vi "is_roi_inside_roi.vi"(8 "Error In":errorcluster, 10 "ROI Outer":T1, 11 "ROI Inner":T1) -> (0 "Error Out":errorcluster, 3 "Inner is inside Outer":bool)   [LabVIEW 2019]
doc: "Determines if one ROI is inside another ROI or not based on their global rectangles."
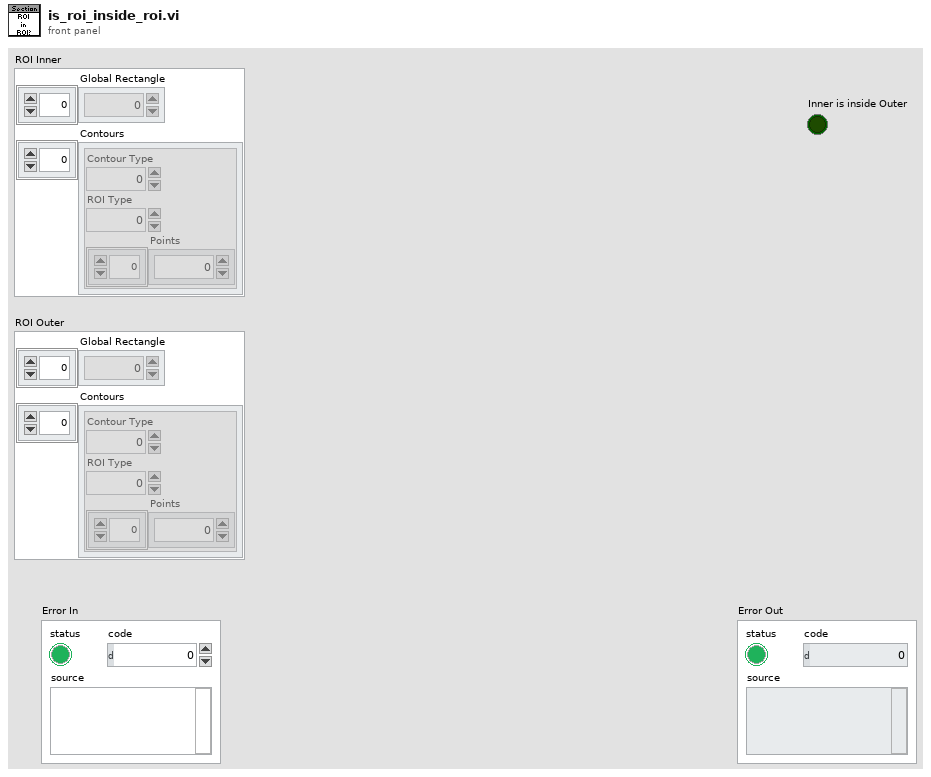
[diagram p1: front panel]
types:
  T1 = cluster{"Global Rectangle":i32[], "Contours":cluster{"Contour Type":u32, "ROI Type":u32, "Points":i32[]}[]}
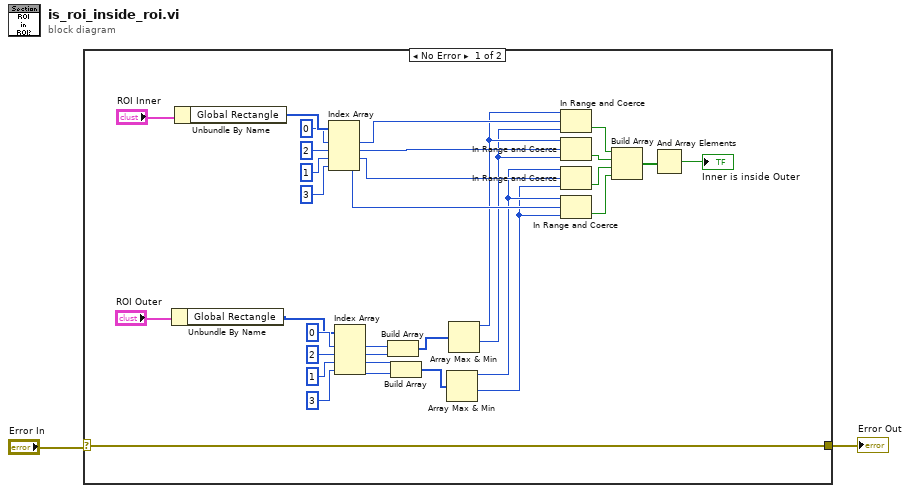
[diagram p0: block diagram]
diagram:
  n1 = case shown="No Error" "Error In" {
    selector: "Error In" -> [w35 w36]
    tunnel: [w35 w36] -> w1
    frame No Error {
      n2 = Unbundle By Name("ROI Outer") -> ("Global Rectangle"=w24:i32[])
      n3 = Unbundle By Name("ROI Inner") -> ("Global Rectangle"=w32:i32[])
      n4 = Index Array(array=w32, index #1=0 ("index"), index #2=2 ("index"), index #3=1 ("index"), index #4=3 ("index")) -> (element #1=w18:i32, element #2=w17:i32, element #3=w16:i32, element #4=w15:i32)
      n5 = Index Array(array=w24, index #1=0 ("index"), index #2=2 ("index"), index #3=1 ("index"), index #4=3 ("index")) -> (element #1=w19:i32, element #2=w22:i32, element #3=w21:i32, element #4=w20:i32)
      n6 = Build Array(w19, w22) -> (w14:i32[])
      n7 = Build Array(w21, w20) -> (w13:i32[])
      n8 = Array Max & Min(array=w13) -> (max value=w10:i32, min value=w9:i32)  [unwired: 2 out]
      n9 = Array Max & Min(array=w14) -> (max value=w12:i32, min value=w11:i32)  [unwired: 2 out]
      n10 = In Range and Coerce(upper limit=w12, x=w18, lower limit=w11) -> (In Range?=w8:bool)  [unwired: 1 out]
      n11 = In Range and Coerce(upper limit=w12, x=w17, lower limit=w11) -> (In Range?=w7:bool)  [unwired: 1 out]
      n12 = In Range and Coerce(upper limit=w10, x=w16, lower limit=w9) -> (In Range?=w6:bool)  [unwired: 1 out]
      n13 = In Range and Coerce(upper limit=w10, x=w15, lower limit=w9) -> (In Range?=w5:bool)  [unwired: 1 out]
      n14 = Build Array(w8, w7, w6, w5) -> (w4:bool[])
      n15 = And Array Elements(Boolean array=w4) -> (logical AND=→"Inner is inside Outer":bool)
    }
    frame Error {
    }
  }
  "Error Out" <- w1
